vi "A Neighbour is Full.vi"(0 "Cell":i32, 5 "Parsed Board":T1, 11 "error in (no error)":errorcluster) -> (4 "Full?":bool, 15 "error out":errorcluster)   [LabVIEW 2014, in "Dragon Tamers.lvlib"]
uses:
  Dragon Tamers.lvlib
  Typedefs/Parsed Board.ctl
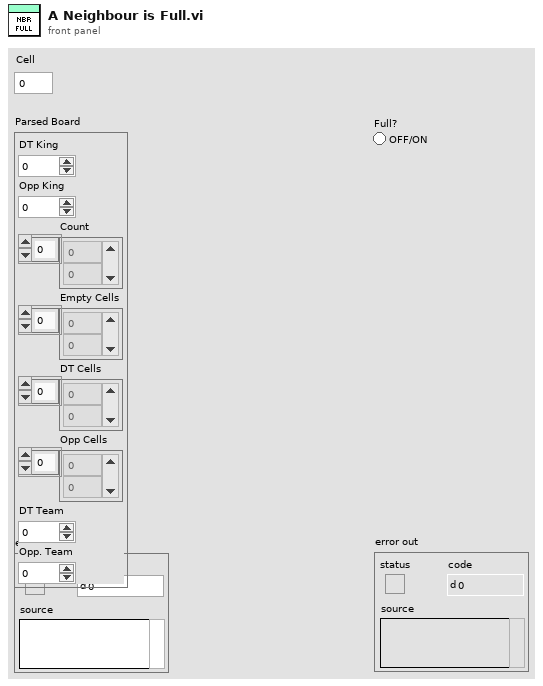
[diagram p1: front panel]
types:
  T1 = typedef "Dragon Tamers.lvlib/Parsed Board.ctl" = cluster{"DT King":i32, "Opp King":i32, "Count":i32[], "Empty Cells":i32[], "DT Cells":i32[], "Opp Cells":i32[], "DT Team":i32, "Opp. Team":i32}
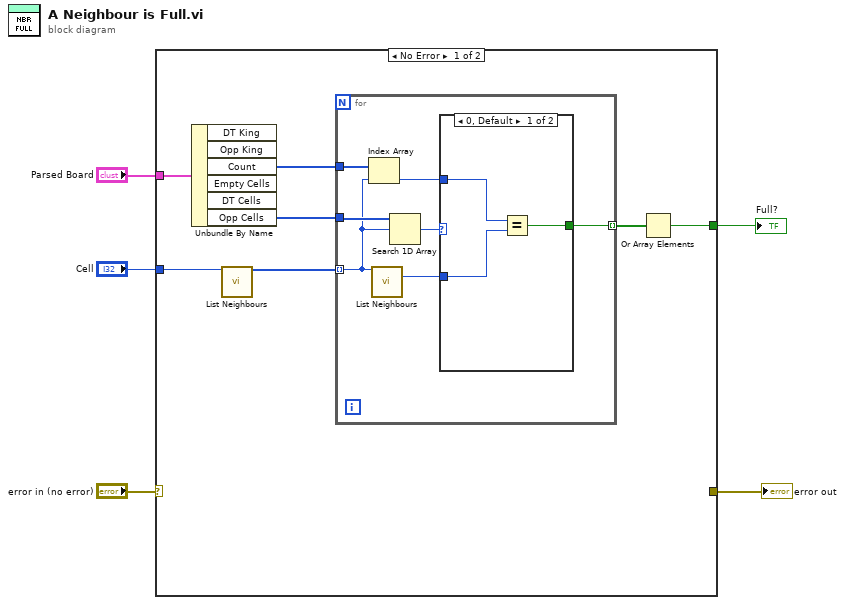
[diagram p0: block diagram]
diagram:
  n1 = case shown="No Error" "error in (no error)" {
    selector: "error in (no error)" -> [_ w23]
    tunnel: [_ w23] -> w4
    tunnel: "Cell" -> [w12 _]
    tunnel: "Parsed Board" -> [w11 _]
    tunnel: [w6 _] -> w1
    frame No Error {
      n2 = Unbundle By Name(w11) -> ("Count"=w9:i32[], "Opp Cells"=w8:i32[])  [unwired: 4 out]
      n3 = call "List Neighbours.vi"("Cell Index"=w12) -> ("Neighbours"=w10:i32[])  [unwired: 12 in, 2 out]
      n4 = for {
        tunnel: w10 -> [w17] mode=indexing
        tunnel: w9 -> [w19]
        tunnel: w8 -> [w18]
        tunnel: [w13] -> w7 mode=indexing
        n5 = Index Array(array=w19, index=w17) -> (element=w15:i32)
        n6 = call "List Neighbours.vi"("Cell Index"=w17) -> ("Max Capacity"=w14:i32)  [unwired: 12 in, 2 out]
        n7 = Search 1D Array(1D array=w18, element=w17) -> (index of element=w16:i32)  [unwired: 1 in]
        n8 = case shown="0, Default" w16 {
          tunnel: w15 -> [w22 _]
          tunnel: w14 -> [w21 _]
          tunnel: [w20 _] -> w13
          frame 0, Default {
            n9 = Equal?(x=w22, y=w21) -> (x = y?=w20:bool)
          }
          frame -1 {
          }
        }
      }
      n10 = Or Array Elements(Boolean array=w7) -> (logical OR=w6:bool)
    }
    frame Error {
    }
  }
  "error out" <- w4
  "Full?" <- w1
